vi "H5Dread (Variant).vi"(4 "Data":variant, 5 "HDF5 File Space (H5S_ALL)":T1, 7 "HDF5 Memory Space":T1, 8 "error in (no error)":errorcluster, 9 "HDF5 Xfer Property List":T1, 10 "HDF5 Type Ref (match data)":T1, 11 "HDF5 Dataset Ref":T1) -> (0 "error out":errorcluster, 1 "Data out":variant, 3 "HDF5 Dataset Ref out":T1)   [LabVIEW 2017]
doc: "Reads data from a dataset into a buffer."
uses:
  <vilib>/UPVI/lvhdf5/library.llb/HDF5 Ref.ctl
  <vilib>/UPVI/lvhdf5/identifier.llb/H5Iget_type.vi
  <vilib>/UPVI/lvhdf5/h5helper.dll
panel:
  # "LVHDF5 Toolkit\nCopyright (c) 2005-2013 by Jason D. Sommerville\nCopyright (c) 2014 by UPVI, LLC.\n\nThis use and distribution of this file is governed by the terms found in \nLICENSE.txt distributed with this toolkit and installed at\n <user.lib>\\_lvhdf5\\LICENSE.txt"
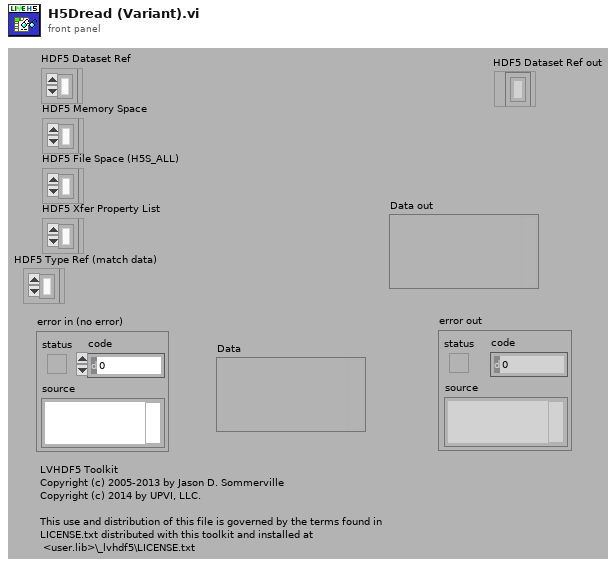
[diagram p1: front panel]
types:
  T1 = typedef "HDF5 Ref.ctl" = refnum<k1>
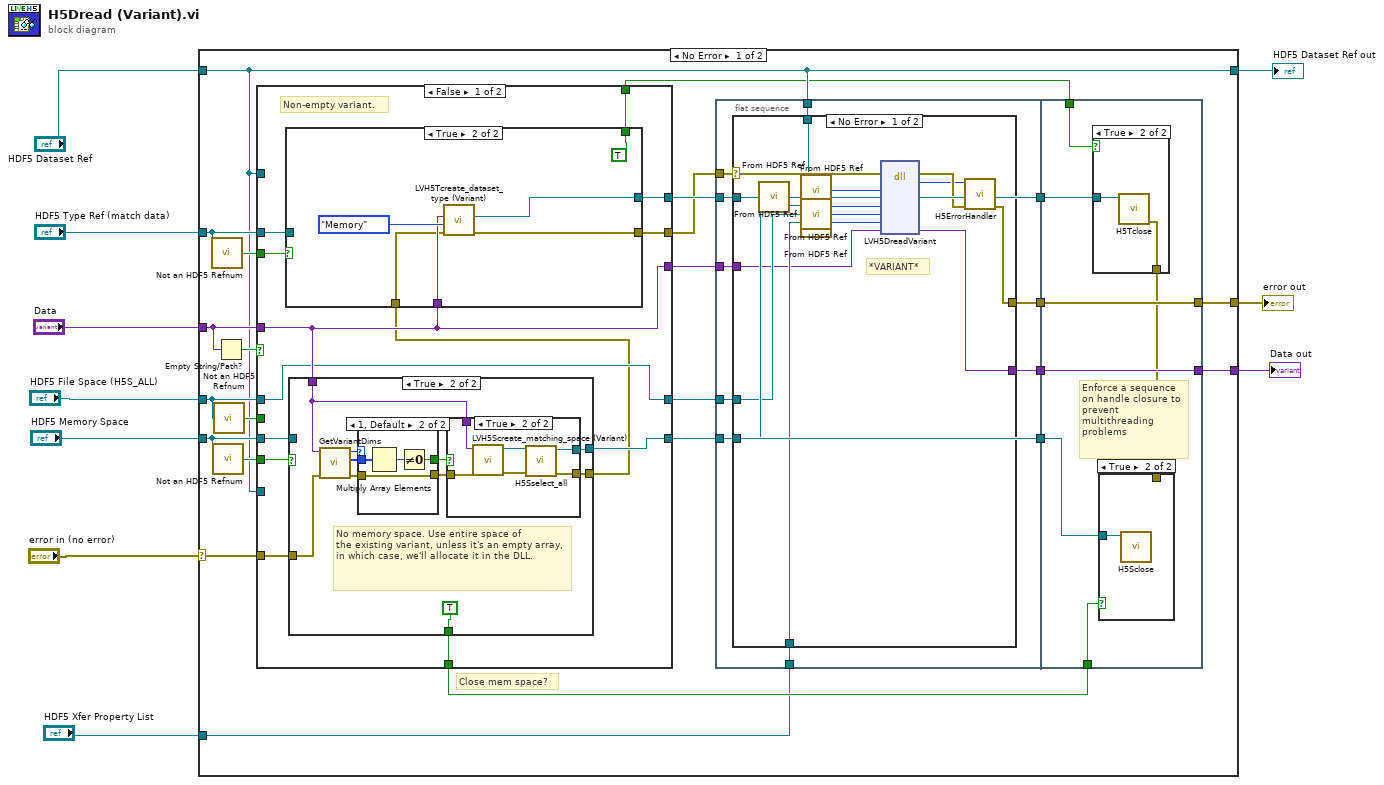
[diagram p0: block diagram]
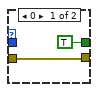
[diagram p4: hidden frame]
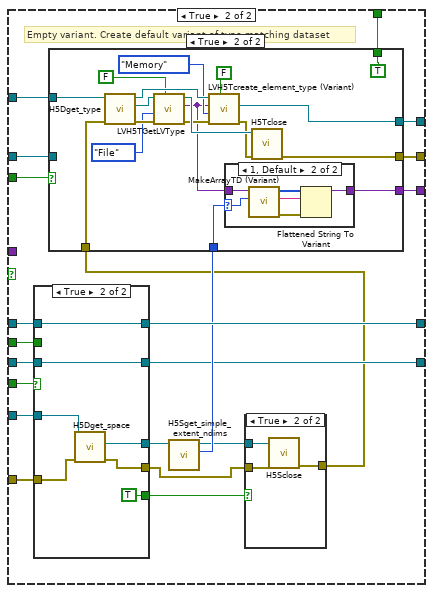
[diagram p6: hidden frame]
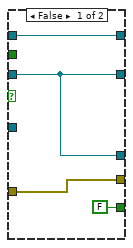
[diagram p8: hidden frame]
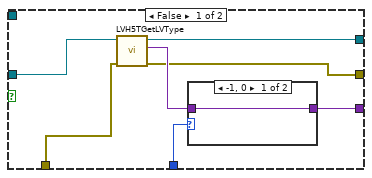
[diagram p9: hidden frame]
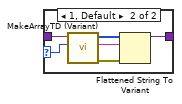
[diagram p10: hidden frame]
diagram:
  n1 = case shown="No Error" "error in (no error)" {
    selector: "error in (no error)" -> [w25 w193]
    tunnel: [w34 w193] -> w3
    tunnel: "HDF5 Dataset Ref" -> [w17 w192]
    tunnel: "HDF5 Xfer Property List" -> [w12 _]
    tunnel: "HDF5 File Space (H5S_ALL)" -> [w23 _]
    tunnel: "HDF5 Memory Space" -> [w28 _]
    tunnel: "Data" -> [w27 _]
    tunnel: "HDF5 Type Ref (match data)" -> [w21 _]
    tunnel: [w32 _] -> w4
    tunnel: [w17 w192] -> w2
    frame No Error {
      # "Close mem space?"
      n2 = call <vilib>:"Not an HDF5 Refnum.vi"("HDF5 Ref"=w21) -> ("Not an HDF5 Refnum"=w26:bool)
      n3 = call <vilib>:"Not an HDF5 Refnum.vi"("HDF5 Ref"=w28) -> ("Not an HDF5 Refnum"=w29:bool)
      n4 = call <vilib>:"Not an HDF5 Refnum.vi"("HDF5 Ref"=w23) -> ("Not an HDF5 Refnum"=w22:bool)
      n5 = Empty String/Path?(string/path=w27) -> (empty?=w30:bool)
      n6 = case shown="False" w30 {
        tunnel: w29 -> [w44 w99]
        tunnel: w28 -> [w36 w98]
        tunnel: w27 -> [w43 _]
        tunnel: w26 -> [w47 w100]
        tunnel: w25 -> [w42 w89]
        tunnel: [w46 w101] -> w24
        tunnel: w23 -> [w40 w97]
        tunnel: w22 -> [_ w96]
        tunnel: w17 -> [_ w95]
        tunnel: [w40 w94] -> w19
        tunnel: [w43 w91] -> w11
        tunnel: w21 -> [w45 w90]
        tunnel: [w39 w88] -> w20
        tunnel: [w37 w84] -> w13
        tunnel: [w41 _] -> w18
        tunnel: w17 -> [_ w82]
        tunnel: [w35 w81] -> w16
        frame False {
          # "Non-empty variant."
          n7 = case shown="True" w44 {
            tunnel: [w49 w57] -> w38
            tunnel: [w48 w58] -> w39
            tunnel: w43 -> [_ w52]
            tunnel: w42 -> [w49 w56]
            tunnel: [_ TRUE] -> w41
            tunnel: w36 -> [w48 _]
            frame False {
              # "Memory space\nspecified.\nSomething in _Data.\nHopefully they work together, but it's out of our hands."
            }
            frame True {
              # "No memory space. Use entire space of \nthe existing variant, unless it's an empty array, in which case, we'll allocate it in the DLL."
              n8 = call <vilib>:"GetVariantDims.vi"("error in (no error)"=w56, "Variant"=w52) -> ("error out"=w53:errorcluster, "Array"=w54:i32[], "rank"=w55:i32)  [unwired: 7 in]
              n9 = case shown="1, Default" w55 {
                tunnel: w54 -> [_ w72]
                tunnel: [TRUE w70] -> w50
                tunnel: [w67 w69] -> w51
                tunnel: w53 -> [w67 w69]
                frame 0 {
                }
                frame 1, Default {
                  n10 = Multiply Array Elements(1:w72) -> (0:w71:i32)
                  n11 = Not Equal To 0?(x=w71) -> (x != 0?=w70:bool)
                }
              }
              n12 = case shown="True" w50 {
                tunnel: [_ w64] -> w58
                tunnel: [w60 w63] -> w57
                tunnel: w52 -> [_ w62]
                tunnel: w51 -> [w60 w61]
                frame False {
                }
                frame True {
                  n13 = call <vilib>:"LVH5Screate_matching_space (Variant).vi"("error in (no error)"=w61, "Data"=w62) -> ("error out"=w66:errorcluster, "HDF5 Dataspace Ref"=w65:T1)  [unwired: 6 in]
                  n14 = call <vilib>:"H5Sselect_all.vi"("error in (no error)"=w66, "HDF5 Space Ref"=w65) -> ("error out"=w63:errorcluster, "HDF5 Ref out"=w64:T1)  [unwired: 6 in]
                }
              }
            }
          }
          n15 = case shown="True" w47 {
            tunnel: w43 -> [_ w79]
            tunnel: [w74 w78] -> w46
            tunnel: w45 -> [w74 _]
            tunnel: w38 -> [w73 w77]
            tunnel: [w73 w76] -> w37
            tunnel: [_ TRUE] -> w35
            frame False {
            }
            frame True {
              n16 = call <vilib>:"LVH5Tcreate_dataset_type (Variant).vi"("error in (no error)"=w77, "Type"=enum16{"File", "Memory"}."Memory", "Data"=w79) -> ("error out"=w76:errorcluster, "HDF5 Type Ref"=w78:T1)  [unwired: 4 in, 3 out]
            }
          }
        }
        frame True {
          # "Empty variant. Create default variant of type matching dataset"
          n17 = case shown="True" w99 {
            tunnel: w98 -> [w107 w111]
            tunnel: w97 -> [w109 w116]
            tunnel: w96 -> [_ _]
            tunnel: w95 -> [_ w112]
            tunnel: [w107 w115] -> w93
            tunnel: [w109 w116] -> w94
            tunnel: w89 -> [w108 w114]
            tunnel: [w108 w113] -> w83
            tunnel: [w107 w111] -> w88
            tunnel: [FALSE TRUE] -> w86
            frame False {
            }
            frame True {
              n18 = call <vilib>:"H5Dget_space.vi"("error in (no error)"=w114, "HDF5 Dataset Ref"=w112) -> ("error out"=w113:errorcluster, "HDF5 Dataspace Ref"=w115:T1)  [unwired: 5 in, 1 out]
            }
          }
          n19 = call <vilib>:"H5Sget_simple_extent_ndims.vi"("HDF5 Space Ref"=w93) -> ("Rank"=w92:i32, "HDF5 Ref out"=w87:T1)  [unwired: 6 in, 1 out]
          n20 = case shown="True" w86 {
            tunnel: w87 -> [_ w105]
            tunnel: w83 -> [w102 w104]
            tunnel: [w102 w103] -> w85
            frame False {
            }
            frame True {
              n21 = call <vilib>:"H5Sclose.vi"("error in (no error)"=w104, "HDF5 Dataspace Ref"=w105) -> ("error out"=w103:errorcluster)  [unwired: 7 in]
            }
          }
          n22 = case shown="True" w100 {
            tunnel: [w120 w143] -> w101
            tunnel: w92 -> [w122 w142]
            tunnel: [w117 w140] -> w91
            tunnel: w90 -> [w121 _]
            tunnel: w85 -> [w119 w139]
            tunnel: [w118 w138] -> w84
            tunnel: w82 -> [_ w137]
            tunnel: [_ TRUE] -> w81
            frame False {
              n23 = call <vilib>:"LVH5TGetLVType.vi"("error in (no error)"=w119, "HDF5 Type Ref"=w121) -> ("error out"=w118:errorcluster, "Data Type"=w123:variant, "HDF5 Type Ref out"=w120:T1)  [unwired: 5 in, 2 out]
              n24 = case shown="-1, 0" w122 {
                selector: w122 -> [_ w130]
                tunnel: w123 -> [w124 w129]
                tunnel: [w124 w125] -> w117
                frame -1, 0 {
                }
                frame 1, Default {
                  n25 = call <vilib>:"MakeArrayTD (Variant).vi"("rank"=w130, "Element type_id"=w129) -> ("error out"=w128:errorcluster, "Default Data"=w127:string, "td"=w126:i16[])  [unwired: 7 in]
                  n26 = Flattened String To Variant(4:w128, 6:w127, 7:w126) -> (3:w125:variant)  [unwired: 1 out]
                }
              }
            }
            frame True {
              n27 = call <vilib>:"H5Dget_type.vi"("error in (no error)"=w139, "HDF5 Dataset Ref"=w137) -> ("error out"=w135:errorcluster, "HDF5 Datatype Ref"=w134:T1, "HDF5 Dataset Ref out"=w145:T1)  [unwired: 5 in]
              n28 = call <vilib>:"LVH5TGetLVType.vi"("Don't use cache"=FALSE, "error in (no error)"=w135, "Type"=enum16{"File", "Memory"}."File", "HDF5 Type Ref"=w134) -> ("error out"=w146:errorcluster, "Data Type"=w141:variant, "HDF5 Type Ref out"=w148:T1)  [unwired: 3 in, 2 out]
              n29 = call <vilib>:"LVH5Tcreate_element_type (Variant).vi"("Don't use cache"=FALSE, "error in (no error)"=w146, "Type"=enum16{"File", "Memory"}."Memory", "Data"=w141, "HDF5 Location Ref"=w145) -> ("error out"=w147:errorcluster, "HDF5 Type Ref"=w143:T1)  [unwired: 2 in, 3 out]
              n30 = case shown="1, Default" w142 {
                selector: w142 -> [_ w155]
                tunnel: w141 -> [w149 w154]
                tunnel: [w149 w150] -> w140
                frame -1, 0 {
                }
                frame 1, Default {
                  n31 = call <vilib>:"MakeArrayTD (Variant).vi"("rank"=w155, "Element type_id"=w154) -> ("error out"=w153:errorcluster, "Default Data"=w152:string, "td"=w151:i16[])  [unwired: 7 in]
                  n32 = Flattened String To Variant(4:w153, 6:w152, 7:w151) -> (3:w150:variant)  [unwired: 1 out]
                }
              }
              n33 = call <vilib>:"H5Tclose.vi"("error in (no error)"=w147, "HDF5 Datatype Ref"=w148) -> ("error out"=w138:errorcluster)  [unwired: 7 in]
            }
          }
        }
      }
      n34 = flat-sequence {
        tunnel: w17 -> [w163]
        tunnel: [w164] -> w33
        tunnel: [w162] -> w31
        tunnel: w13 -> [w161]
        tunnel: w24 -> [w159]
        tunnel: w20 -> [w158]
        tunnel: w19 -> [w160]
        tunnel: [w159] -> w15
        tunnel: [w158] -> w14
        tunnel: w12 -> [w157]
        tunnel: w11 -> [w156]
        tunnel: [w188] -> w34
        tunnel: w33 -> [w188]
        tunnel: [w187] -> w32
        tunnel: w31 -> [w187]
        tunnel: w18 -> [w186]
        tunnel: w16 -> [w185]
        tunnel: w15 -> [w184]
        tunnel: w14 -> [w183]
        frame #0 {
          n35 = case shown="No Error" w161 {
            selector: w161 -> [w172 w181]
            tunnel: w163 -> [w171 _]
            tunnel: [w175 w181] -> w164
            tunnel: [w170 _] -> w162
            tunnel: w159 -> [w169 _]
            tunnel: w158 -> [w168 _]
            tunnel: w160 -> [w167 _]
            tunnel: w157 -> [w166 _]
            tunnel: w156 -> [w165 _]
            frame No Error {
              # "*VARIANT*"
              n36 = call <vilib>:"From HDF5 Ref.vi"("HDF5 Ref"=w169) -> ("I32"=w176:i32)
              n37 = call <vilib>:"From HDF5 Ref.vi"("HDF5 Ref"=w171) -> ("I32"=w179:i32)
              n38 = call <vilib>:"From HDF5 Ref.vi"("HDF5 Ref"=w168) -> ("I32"=w173:i32)
              n39 = call <vilib>:"From HDF5 Ref.vi"("HDF5 Ref"=w167) -> ("I32"=w178:i32)
              n40 = call <vilib>:"From HDF5 Ref.vi"("HDF5 Ref"=w166) -> ("I32"=w177:i32)
              n41 = dll-call lib="C:/Program Files/National Instruments/LabVIEW 2017/vi.lib/UPVI/lvhdf5/h5helper.dll" fn="LVH5DreadVariant"(error in=w172, "dataset_id"=w179, "mem_type_id"=w176, "mem_space_id"=w173, "file_space_id"=w178, "xfer_plist_id"=w177, "plvvar"=w165) -> (error out=w180:errorcluster, "return type"=w174:i32, "plvvar"=w170:variant)  [unwired: 7 in, 1 out]
              n42 = call <vilib>:"H5ErrorHandler.vi"("error in (no error)"=w180, "herr_t"=w174) -> ("error out"=w175:errorcluster)  [unwired: 3 in, 4 out]
            }
            frame Error {
            }
          }
        }
        frame #1 {
          # "Enforce a sequence on handle closure to prevent multithreading problems"
          n43 = case shown="True" w185 {
            tunnel: w184 -> [_ w191]
            tunnel: [_ w190] -> w182
            frame False {
            }
            frame True {
              n44 = call <vilib>:"H5Tclose.vi"("HDF5 Datatype Ref"=w191) -> ("error out"=w190:errorcluster)  [unwired: 8 in]
            }
          }
          n45 = case shown="True" w186 {
            tunnel: w183 -> [_ w189]
            tunnel: w182 -> [_ _]
            frame False {
            }
            frame True {
              n46 = call <vilib>:"H5Sclose.vi"("HDF5 Dataspace Ref"=w189) -> ()  [unwired: 8 in, 1 out]
            }
          }
        }
      }
    }
    frame Error {
    }
  }
  "error out" <- w3
  "HDF5 Dataset Ref out" <- w2
  "Data out" <- w4
